vi "opse_project.vi"() -> ()   [LabVIEW 2018]
uses:
  <vilib>/DAQmx/write.llb/DAQmx Write (Digital U8 1Chan 1Samp).vi
  <vilib>/DAQmx/create/channels.llb/DAQmx Create Channel (DO-Digital Output).vi
  <vilib>/DAQmx/miscellaneous.llb/DAQmx Fill In Error Info.vi
panel:
  out "max corrsponding to graph":dbl=3.1083844580777065
  in  "distance from lens to end of scale":dbl=5.1
  in  "Initial length from lens":dbl=8.0
  out "Motor/DAQ error":errorcluster
  out "Lockin Error":errorcluster
  out "focal length":dbl=7.591615541922293
  out "XY Graph":cluster{"Y":dbl[], "Y":dbl[]}[](graph)=[{"Y"=[0.0, 0.032719836400818, 0.065439672801636, 0.09815950920245399, 0.130879345603272, 0.16359918200409, 0.19631901840490798, 0.22903885480572594, 0.26175869120654394, 0.29447852760736193, 0.3271983640081799, 0.3599182004089979, 0.39263803680981585, 0.42535787321063384, 0.45807770961145183, 0.4907975460122698, 0.5235173824130878, 0.5562372188139058, 0.5889570552147239, 0.6216768916155418, 0.65439672801636, 0.6871165644171779, 0.719836400817996, 0.752556237218814, 0.7852760736196321, 0.8179959100204501, 0.8507157464212682, 0.8834355828220862, 0.9161554192229043, 0.9488752556237223, 0.9815950920245403, 1.0143149284253583, 1.0470347648261764, 1.0797546012269945, 1.1124744376278126, 1.1451942740286305, 1.1779141104294486, 1.2106339468302667, 1.2433537832310848, 1.2760736196319027, 1.3087934560327208, 1.341513292433539, 1.374233128834357, 1.4069529652351749, 1.439672801635993, 1.472392638036811, 1.505112474437629, 1.537832310838447, 1.5705521472392652, 1.6032719836400833, 1.6359918200409012, 1.6687116564417193, 1.7014314928425374, 1.7341513292433555, 1.7668711656441733, 1.7995910020449915, 1.8323108384458096, 1.8650306748466277, 1.8977505112474455, 1.9304703476482636, 1.9631901840490817, 1.9959100204498996, 2.028629856850718, 2.0613496932515356, 2.0940695296523537, 2.126789366053172, 2.15950920245399, 2.1922290388548076, 2.2249488752556257, 2.2576687116564433, 2.290388548057261, 2.323108384458079, 2.3558282208588968, 2.3885480572597144, 2.4212678936605325, 2.45398773006135, 2.486707566462168, 2.519427402862986, 2.5521472392638036, 2.5848670756646213, 2.6175869120654394, 2.650306748466257, 2.6830265848670747, 2.715746421267893, 2.7484662576687104, 2.781186094069528, 2.813905930470346, 2.846625766871164, 2.8793456032719815, 2.9120654396727996, 2.9447852760736173, 2.977505112474435, 3.010224948875253, 3.0429447852760707, 3.0756646216768884, 3.1083844580777065, 3.141104294478524, 3.173824130879342, 3.20654396728016, 3.2392638036809775, 3.271983640081795, 3.3047034764826133, 3.337423312883431, 3.3701431492842486, 3.4028629856850667, 3.4355828220858844, 3.468302658486702, 3.50102249488752, 3.533742331288338, 3.5664621676891555, 3.5991820040899736, 3.6319018404907912, 3.664621676891609, 3.697341513292427, 3.7300613496932447, 3.7627811860940623, 3.7955010224948804, 3.828220858895698, 3.8609406952965157, 3.893660531697334, 3.9263803680981515, 3.959100204498969, 3.9918200408997873, 4.024539877300605, 4.057259713701423, 4.089979550102241, 4.122699386503059, 4.155419222903876, 4.188139059304694, 4.220858895705512, 4.253578732106329, 4.2862985685071475, 4.319018404907966, 4.351738241308784, 4.384458077709602, 4.417177914110421, 4.449897750511239, 4.482617586912057, 4.515337423312875, 4.548057259713693, 4.580777096114512, 4.61349693251533, 4.646216768916148, 4.6789366053169665, 4.711656441717785, 4.744376278118604, 4.777096114519422], "Y"=[-0.04, -0.03, -0.035, -0.04, -0.04, -0.03, -0.024999999999999998, -0.03, -0.015, -0.015, -0.0, -0.01, 0.01, -0.035, -0.01, 0.015, 0.049999999999999996, 0.035, -0.055, 0.075, 0.015, 0.005, 0.035, 0.08499999999999999, 0.065, 0.035, 0.015, -0.01, 0.005, -0.005, 0.035, -0.015, 0.08499999999999999, 0.065, 0.049999999999999996, 0.049999999999999996, 0.03, 0.09999999999999999, 0.01, -0.005, 0.035, 0.08499999999999999, 0.049999999999999996, 0.06, 0.075, 0.01, 0.055, 0.055, 0.024999999999999998, 0.075, 0.08499999999999999, -0.005, 0.06, 0.08499999999999999, -0.005, 0.035, 0.08499999999999999, 0.08499999999999999, 0.09, 0.11, 0.049999999999999996, 0.065, 0.075, 0.08499999999999999, 0.055, 0.01, 0.065, 0.06, -0.205, -0.03, -0.0, -0.11, -0.22499999999999998, -0.31, -0.24, -0.435, -0.38, -0.31, -0.005, 0.03, 0.03, 0.024999999999999998, 0.024999999999999998, 0.01, -1.7, -0.08499999999999999, -0.049999999999999996, -0.049999999999999996, -0.049999999999999996, -0.049999999999999996, -0.055, -0.04, -0.035, -0.035, -4.4750000000000005, 8.42, -2.8200000000000003, -3.3249999999999997, -7.57, -9.735000000000001, -9.745000000000001, -6.915, -6.45, -9.965, -10.07, -9.595, -3.745, -2.835, -1.675, -0.7250000000000001, -0.25, -0.215, -0.355, -0.45999999999999996, -1.0150000000000001, -1.085, -1.175, -2.525, -4.1049999999999995, -4.655, -7.725, -6.645, -0.615, -4.735, -7.515, -8.025, -8.015, -7.8, -4.865, -7.425, -7.705, -7.49, -7.015, -6.38, -2.8449999999999998, -4.595, -6.145, -1.6700000000000002, -0.035, 0.035, -0.135, -0.04, -0.035, -0.98, -0.28, -1.105, -0.8150000000000001]}]
  out "Distance":dbl[](array[numeric])=[0.0, 0.032719836400818, 0.065439672801636, 0.09815950920245399, 0.130879345603272, 0.16359918200409, 0.19631901840490798, 0.22903885480572594, 0.26175869120654394, 0.29447852760736193, 0.3271983640081799, 0.3599182004089979, 0.39263803680981585, 0.42535787321063384, 0.45807770961145183, 0.4907975460122698, 0.5235173824130878, 0.5562372188139058, 0.5889570552147239, 0.6216768916155418, 0.65439672801636, 0.6871165644171779, 0.719836400817996, 0.752556237218814, 0.7852760736196321, 0.8179959100204501, 0.8507157464212682, 0.8834355828220862, 0.9161554192229043, 0.9488752556237223, 0.9815950920245403, 1.0143149284253583, 1.0470347648261764, 1.0797546012269945, 1.1124744376278126, 1.1451942740286305, 1.1779141104294486, 1.2106339468302667, 1.2433537832310848, 1.2760736196319027, 1.3087934560327208, 1.341513292433539, 1.374233128834357, 1.4069529652351749, 1.439672801635993, 1.472392638036811, 1.505112474437629, 1.537832310838447, 1.5705521472392652, 1.6032719836400833, 1.6359918200409012, 1.6687116564417193, 1.7014314928425374, 1.7341513292433555, 1.7668711656441733, 1.7995910020449915, 1.8323108384458096, 1.8650306748466277, 1.8977505112474455, 1.9304703476482636, 1.9631901840490817, 1.9959100204498996, 2.028629856850718, 2.0613496932515356, 2.0940695296523537, 2.126789366053172, 2.15950920245399, 2.1922290388548076, 2.2249488752556257, 2.2576687116564433, 2.290388548057261, 2.323108384458079, 2.3558282208588968, 2.3885480572597144, 2.4212678936605325, 2.45398773006135, 2.486707566462168, 2.519427402862986, 2.5521472392638036, 2.5848670756646213, 2.6175869120654394, 2.650306748466257, 2.6830265848670747, 2.715746421267893, 2.7484662576687104, 2.781186094069528, 2.813905930470346, 2.846625766871164, 2.8793456032719815, 2.9120654396727996, 2.9447852760736173, 2.977505112474435, 3.010224948875253, 3.0429447852760707, 3.0756646216768884, 3.1083844580777065, 3.141104294478524, 3.173824130879342, 3.20654396728016, 3.2392638036809775, 3.271983640081795, 3.3047034764826133, 3.337423312883431, 3.3701431492842486, 3.4028629856850667, 3.4355828220858844, 3.468302658486702, 3.50102249488752, 3.533742331288338, 3.5664621676891555, 3.5991820040899736, 3.6319018404907912, 3.664621676891609, 3.697341513292427, 3.7300613496932447, 3.7627811860940623, 3.7955010224948804, 3.828220858895698, 3.8609406952965157, 3.893660531697334, 3.9263803680981515, 3.959100204498969, 3.9918200408997873, 4.024539877300605, 4.057259713701423, 4.089979550102241, 4.122699386503059, 4.155419222903876, 4.188139059304694, 4.220858895705512, 4.253578732106329, 4.2862985685071475, 4.319018404907966, 4.351738241308784, 4.384458077709602, 4.417177914110421, 4.449897750511239, 4.482617586912057, 4.515337423312875, 4.548057259713693, 4.580777096114512, 4.61349693251533, 4.646216768916148, 4.6789366053169665, 4.711656441717785, 4.744376278118604, 4.777096114519422]
  out "Intensity":dbl[](array[numeric])=[-0.04, -0.03, -0.035, -0.04, -0.04, -0.03, -0.024999999999999998, -0.03, -0.015, -0.015, -0.0, -0.01, 0.01, -0.035, -0.01, 0.015, 0.049999999999999996, 0.035, -0.055, 0.075, 0.015, 0.005, 0.035, 0.08499999999999999, 0.065, 0.035, 0.015, -0.01, 0.005, -0.005, 0.035, -0.015, 0.08499999999999999, 0.065, 0.049999999999999996, 0.049999999999999996, 0.03, 0.09999999999999999, 0.01, -0.005, 0.035, 0.08499999999999999, 0.049999999999999996, 0.06, 0.075, 0.01, 0.055, 0.055, 0.024999999999999998, 0.075, 0.08499999999999999, -0.005, 0.06, 0.08499999999999999, -0.005, 0.035, 0.08499999999999999, 0.08499999999999999, 0.09, 0.11, 0.049999999999999996, 0.065, 0.075, 0.08499999999999999, 0.055, 0.01, 0.065, 0.06, -0.205, -0.03, -0.0, -0.11, -0.22499999999999998, -0.31, -0.24, -0.435, -0.38, -0.31, -0.005, 0.03, 0.03, 0.024999999999999998, 0.024999999999999998, 0.01, -1.7, -0.08499999999999999, -0.049999999999999996, -0.049999999999999996, -0.049999999999999996, -0.049999999999999996, -0.055, -0.04, -0.035, -0.035, -4.4750000000000005, 8.42, -2.8200000000000003, -3.3249999999999997, -7.57, -9.735000000000001, -9.745000000000001, -6.915, -6.45, -9.965, -10.07, -9.595, -3.745, -2.835, -1.675, -0.7250000000000001, -0.25, -0.215, -0.355, -0.45999999999999996, -1.0150000000000001, -1.085, -1.175, -2.525, -4.1049999999999995, -4.655, -7.725, -6.645, -0.615, -4.735, -7.515, -8.025, -8.015, -7.8, -4.865, -7.425, -7.705, -7.49, -7.015, -6.38, -2.8449999999999998, -4.595, -6.145, -1.6700000000000002, -0.035, 0.035, -0.135, -0.04, -0.035, -0.98, -0.28, -1.105, -0.8150000000000001]
  in  "address":tag="Dev1/port0/line0:7"
  in  "Speed":u32(slide)=163 scale=0.0..1000.0
  in  "Motor Step/Direction":u16(ring)=1 items=["Half Step Forward", "Full Step Forward", "Half Step Backward", "Full Step Backward"]
  in  "stop":bool
  # "Welcome! This is an automated program used to measure the focal length of a lens"
  # "Results:"
  # "inches"
  # "inches"
  # "inches"
  # "Motor Controls:"
  # "Error Messages"
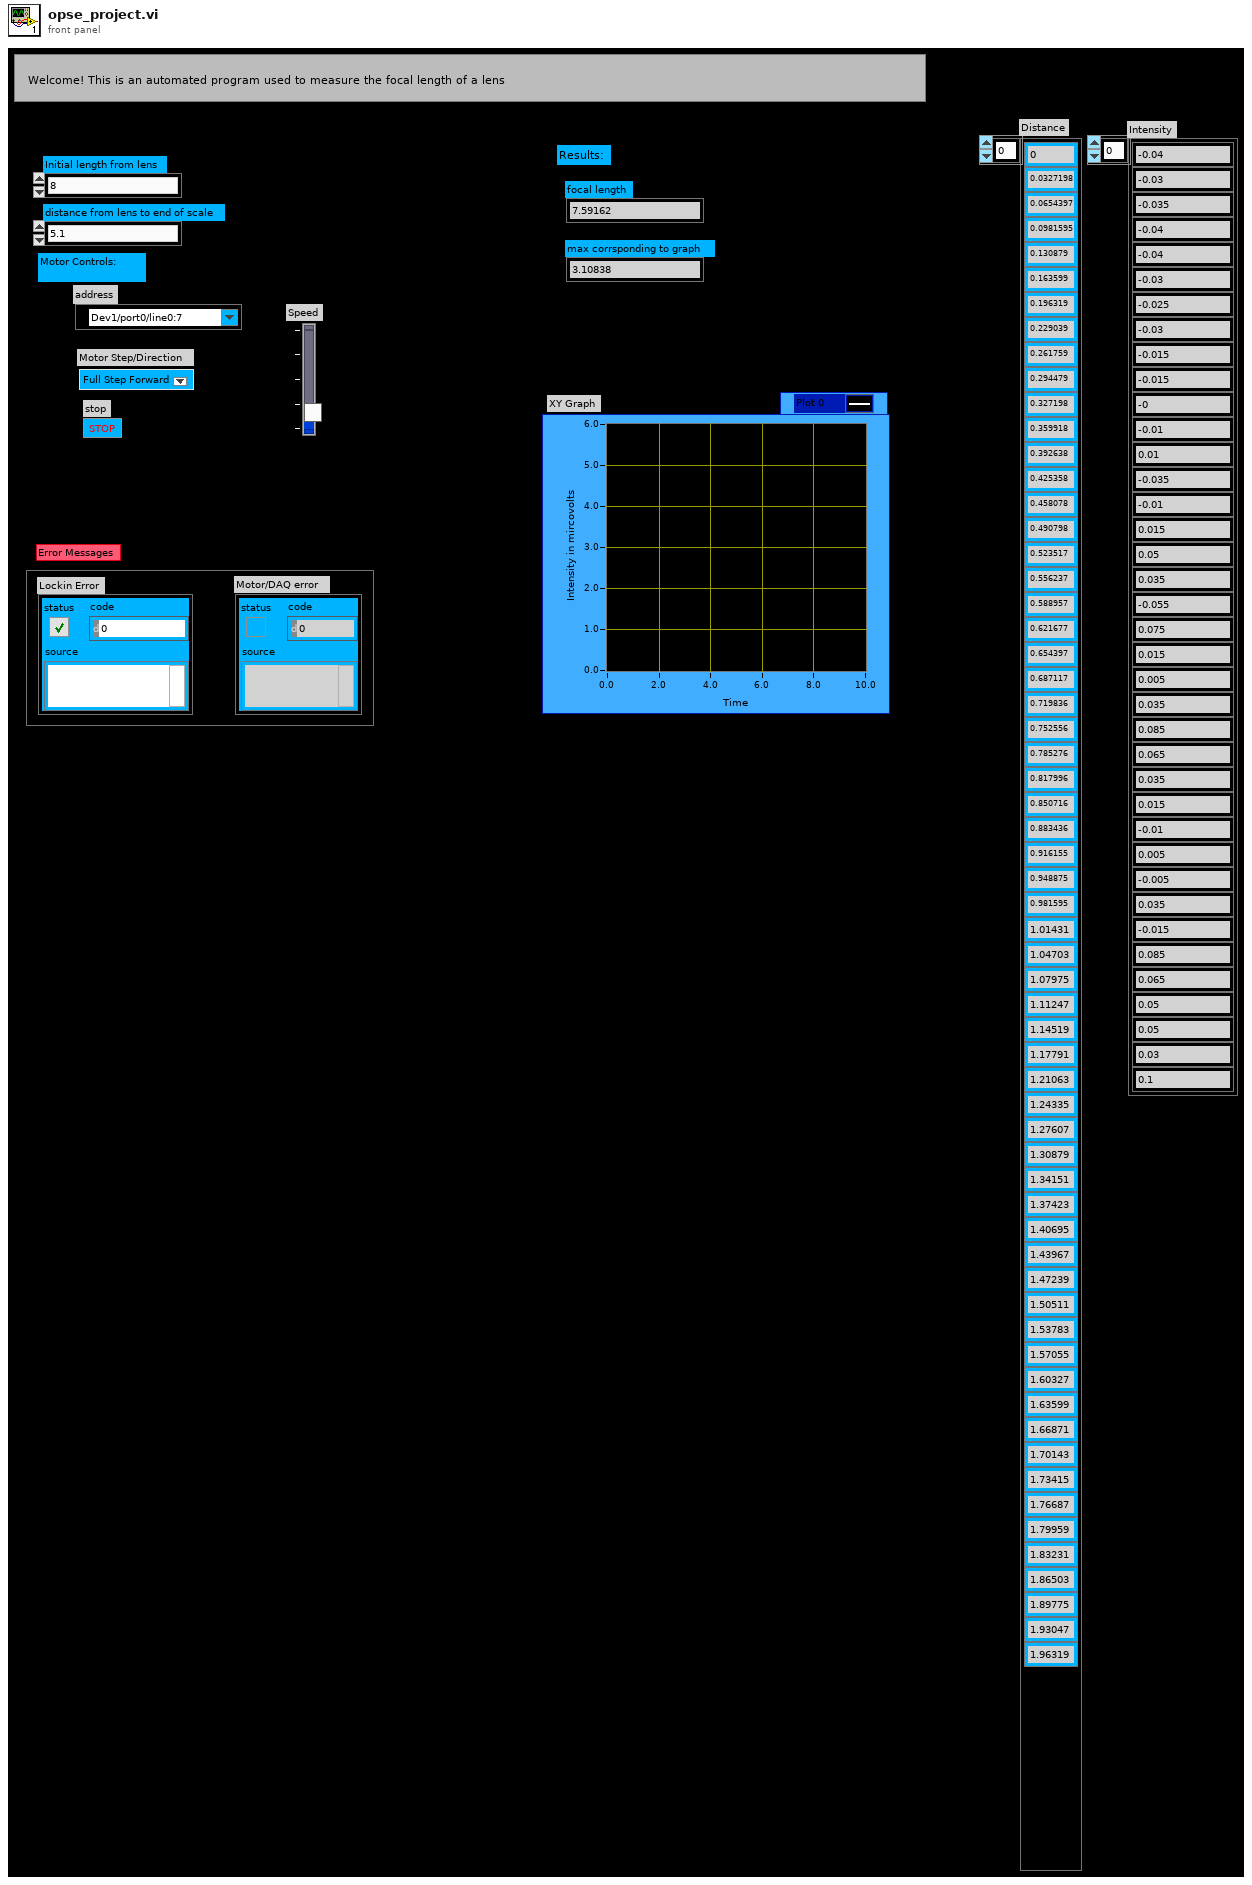
[diagram p1: front panel]
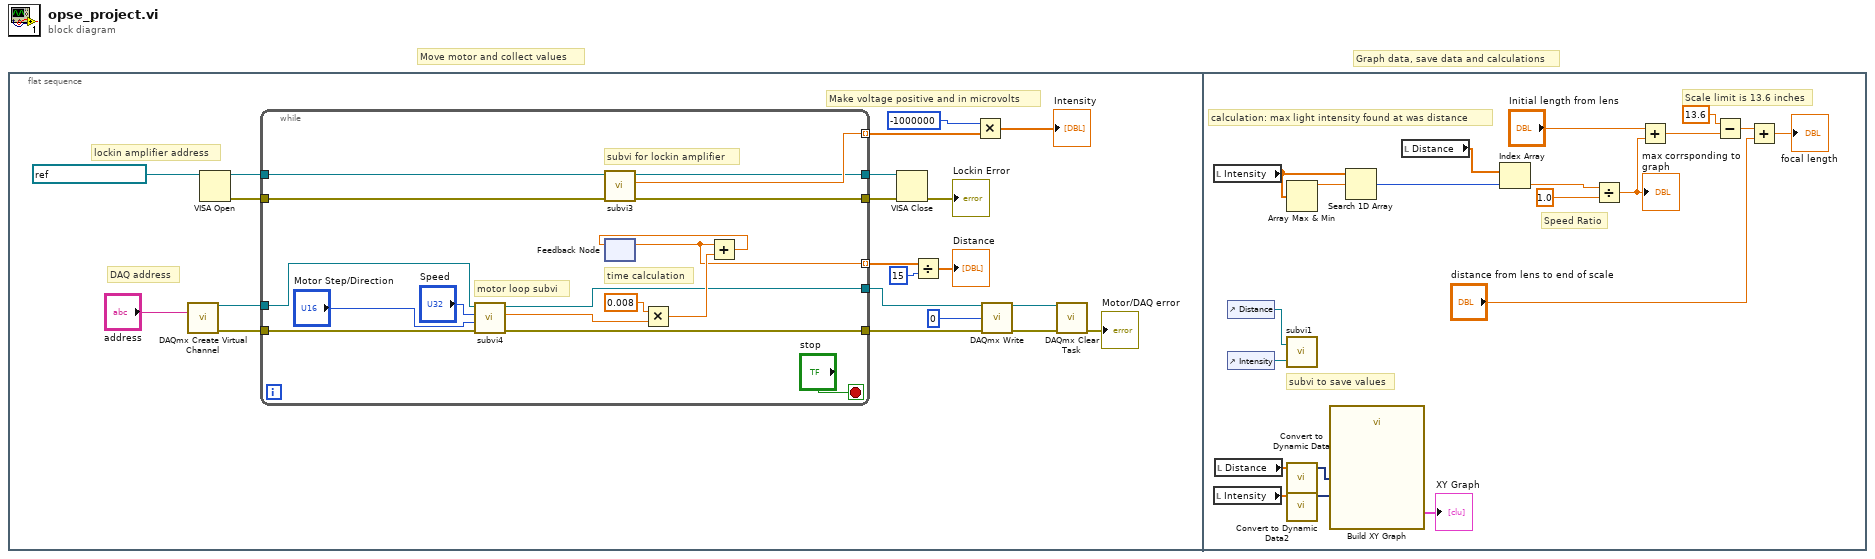
[diagram p0: block diagram]
diagram:
  # "Graph data, save data and calculations"
  # "Move motor and collect values"
  n1 = flat-sequence {
    frame #0 {
      # "Make voltage positive and in microvolts"
      # "DAQ address"
      # "lockin amplifier address"
      n2 = call-poly <vilib>:"DAQmx Create Virtual Channel.vi"("lines"="address") -> ("task out"=w20:refnum<k21>, "error out"=w21:errorcluster)  [unwired: 13 in]
      n3 = VISA Open(VISA resource name=refnum<visa-resource-name> "GPIB0::23::INSTR") -> (VISA resource name=w14:refnum<visa-resource-name>, error out=w12:errorcluster)  [unwired: 4 in]
      n4 = while {
        tunnel: w21 -> [w37]
        tunnel: w20 -> [w36]
        tunnel: [w35] -> w6 mode=indexing
        tunnel: [w24] -> w3 mode=indexing
        tunnel: [w31] -> w18
        tunnel: [w30] -> w16
        tunnel: w14 -> [w29]
        tunnel: [w28] -> w13
        tunnel: w12 -> [w27]
        tunnel: [w26] -> w11
        stop <- "stop" stop-if-true
        # "motor loop subvi"
        # "subvi for lockin amplifier"
        # "time calculation"
        n5 = call "subvi4.vi"("error in (no error)"=w37, "Motor Step/Direction"="Motor Step/Direction", "Speed"="Speed", "Refnum in"=w36) -> ("error out"=w31:errorcluster, "Numeric"=w33:dbl, "Refnum out"=w30:refnum<k21>)  [unwired: 5 in]
        n6 = call "subvi3.vi"("error in (no error)"=w27, "VISA Refnum in"=w29) -> ("error out"=w26:errorcluster, "Numeric"=w35:dbl, "VISA Refnum out"=w28:refnum<visa-resource-name>)  [unwired: 7 in]
        n7 = feedback #1() -> (w24:dbl)  [unwired: 1 in]
        n8 = Multiply(x=0.008, y=w33) -> (x*y=w32:dbl)
        n9 = Add(x=w24, y=w32) -> (x+y=w25:dbl)
        n10 = feedback-in #1(w25) -> ()
      }
      n11 = VISA Close(VISA resource name=w13, error in (no error)=w11) -> (error out=→"Lockin Error":errorcluster)
      n12 = Divide(x=w3, y=15) -> (x/y=→"Distance":dbl[])
      n13 = Multiply(x=-1000000, y=w6) -> (x*y=→"Intensity":dbl[])
      n14 = call-poly <vilib>:"DAQmx Write.vi"("task/channels in"=w16, "data"=0, "error in"=w18) -> ("task out"=w10:refnum<k21>, "error out"=w9:errorcluster)  [unwired: 10 in, 1 out]
      n15 = call <vilib>:"DAQmx Clear Task.vi"("task in"=w10, "error in"=w9) -> ("error out"=→"Motor/DAQ error":errorcluster)  [unwired: 13 in]
    }
    frame #1 {
      # "Scale limit is 13.6 inches"
      # "calculation: max light intensity found at was distance"
      # "subvi to save values"
      # "Speed Ratio"
      n16 = local read "Intensity"() -> (w52:dbl[])
      n17 = local read "Intensity"() -> (w57:dbl[])
      n18 = local read "Distance"() -> (w55:dbl[])
      n19 = control-ref of="Distance"() -> (w47:refnum<vi>)
      n20 = control-ref of="Intensity"() -> (w46:refnum<vi>)
      n21 = Array Max & Min(array=w52) -> (max value=w53:dbl)  [unwired: 3 out]
      n22 = call "subvi1.vi"("reference"=w46, "Array in"=w47) -> ()  [unwired: 2 in]
      n23 = call "Convert to Dynamic Data"("Array"=w55) -> ("Dynamic Data Type"=w56:dynamicdata)  [unwired: 3 in]
      n24 = call "Convert to Dynamic Data2"("Array"=w57) -> ("Dynamic Data Type"=w58:dynamicdata)  [unwired: 3 in]
      n25 = call "Build XY Graph"("Y Input"=w58, "X Input"=w56) -> ("XY Graph"=→"XY Graph":cluster{"X":dbl[], "Y":dbl[]}[])  [unwired: 8 in, 1 out]
      n26 = Search 1D Array(1D array=w52, element=w53) -> (index of element=w51:i32)  [unwired: 1 in]
      n27 = local read "Distance"() -> (w50:dbl[])
      n28 = Index Array(array=w50, index=w51) -> (element=w49:dbl)
      n29 = Divide(x=w49, y=1.0) -> (x/y=w39:dbl)
      "max corrsponding to graph" <- w39
      n30 = Add(x="Initial length from lens", y=w39) -> (x+y=w43:dbl)
      n31 = Subtract(x=13.6, y=w43) -> (x-y=w42:dbl)
      n32 = Add(x=w42, y="distance from lens to end of scale") -> (x+y=→"focal length":dbl)
    }
  }
